vi "demo1.vi"() -> ()   [LabVIEW 2012]
panel:
  in  "Numerisch 3":dbl
  in  "Numerisch 2":dbl
  in  "Numerisch":dbl
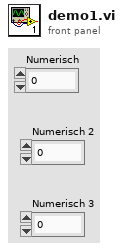
[diagram p1: front panel]
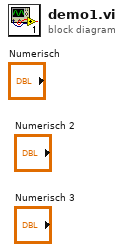
[diagram p0: block diagram]
diagram:
